vi "unflattenFromString.vi"(8 "error in (no error)":errorcluster, 10 "binary string":string, 11 "Task Outputs in":refnum<class "Task Outputs.lvclass">) -> (0 "error out":errorcluster, 3 "Task Outputs out":refnum<class "Task Outputs.lvclass">)   [LabVIEW 2017, in "Message Interface.lvlib" / "Task Outputs.lvclass"]
uses:
  Task Outputs.lvclass
  C:/Users/Public/Documents/wc/BuildFarm/src/LabVIEW/vi.lib/BenjaminR/Build Farm/Classes/Message Interface/Status/Status.lvclass
  Status/Status.lvclass/Status.ctl
  Status/Read Item Name.vi
  Status/Write Item Name.vi
  Status/Status.lvclass
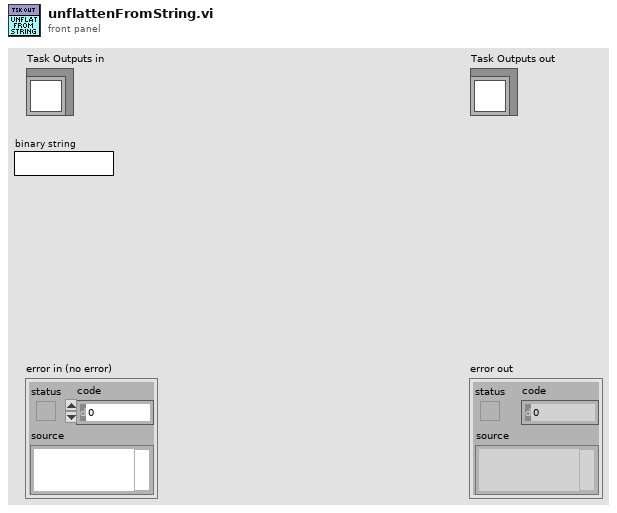
[diagram p1: front panel]
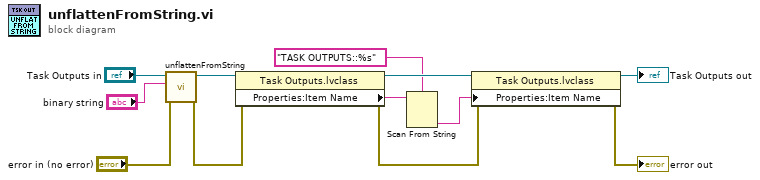
[diagram p0: block diagram]
diagram:
  n1 = call-parent "unflattenFromString.vi"("error in (no error)"="error in (no error)", "binary string"="binary string", "iMessage in"="Task Outputs in") -> ("error out"=w4:errorcluster, "iMessage out"=w6:refnum<class "Task Outputs.lvclass">)  [unwired: 7 in]
  n2 = property class="Task Outputs.lvclass"(reference=w6, error in=w4) -> (reference out=w9:refnum<class "Task Outputs.lvclass">, error out=w2:errorcluster, "Properties:Item Name"=w8:string)
  n3 = Scan From String(format string="TASK OUTPUTS::%s" ("string"), input string=w8) -> (output 1=w1:string)  [unwired: 3 in, 3 out]
  n4 = property class="Task Outputs.lvclass"(reference=w9, error in=w2, "Properties:Item Name"=w1) -> (reference out=→"Task Outputs out":refnum<class "Task Outputs.lvclass">, error out=→"error out":errorcluster)
